vi "Write Visa Com Port 1.vi"(8 "error in (no error)":errorcluster, 10 "Visa Com Port":string, 11 "Serial Device in":refnum<class "Serial Device.lvclass">) -> (0 "error out":errorcluster, 3 "Serial Device out":refnum<class "Serial Device.lvclass">)   [LabVIEW 2020, in "Serial Device.lvclass"]
uses:
  Serial Device.lvclass
  Serial Device.lvclass/Serial Device.ctl
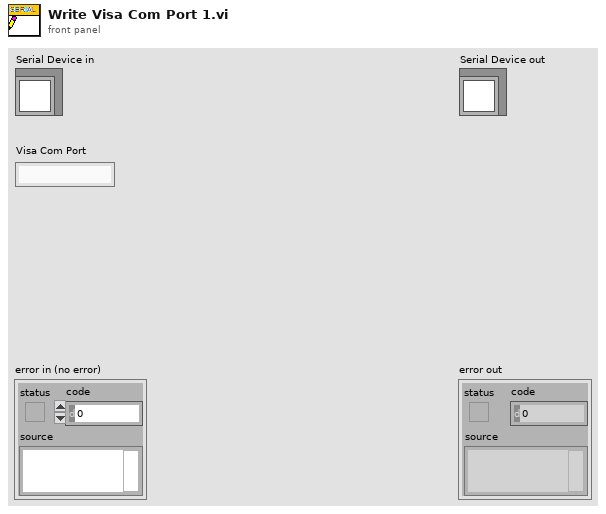
[diagram p1: front panel]
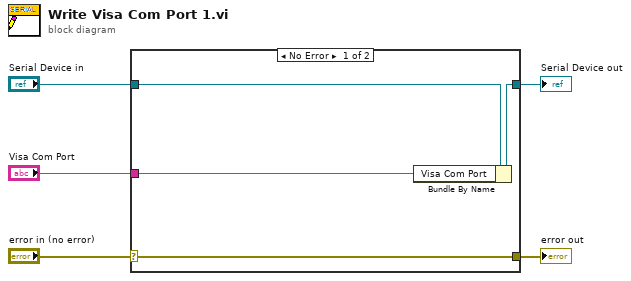
[diagram p0: block diagram]
diagram:
  n1 = case shown="No Error" "error in (no error)" {
    selector: "error in (no error)" -> [w9 w10]
    tunnel: [w9 w10] -> w4
    tunnel: [w7 w11] -> w2
    tunnel: "Serial Device in" -> [w8 w11]
    tunnel: "Visa Com Port" -> [w6 _]
    frame No Error {
      n2 = Bundle By Name(cluster=w8, "Visa Com Port"=w6) -> (w7:refnum<class "Serial Device.lvclass">)
    }
    frame Error {
    }
  }
  "error out" <- w4
  "Serial Device out" <- w2
